vi "mathscrip.vi"(0 "image path":path, 1 "threshoulds array":dbl[](array[numeric]), 5 "error in":errorcluster) -> (12 "imgout":dbl[][](array[numeric]), 13 "error out":errorcluster, 14 "defect ratio 2":dbl, 15 "defect ratio1":dbl, 16 "damage points 2":dbl[][](array[numeric]), 17 "damage points":dbl[][](array[numeric]), 18 "defect type":dbl, 19 "frame statue":dbl)   [LabVIEW 2019]
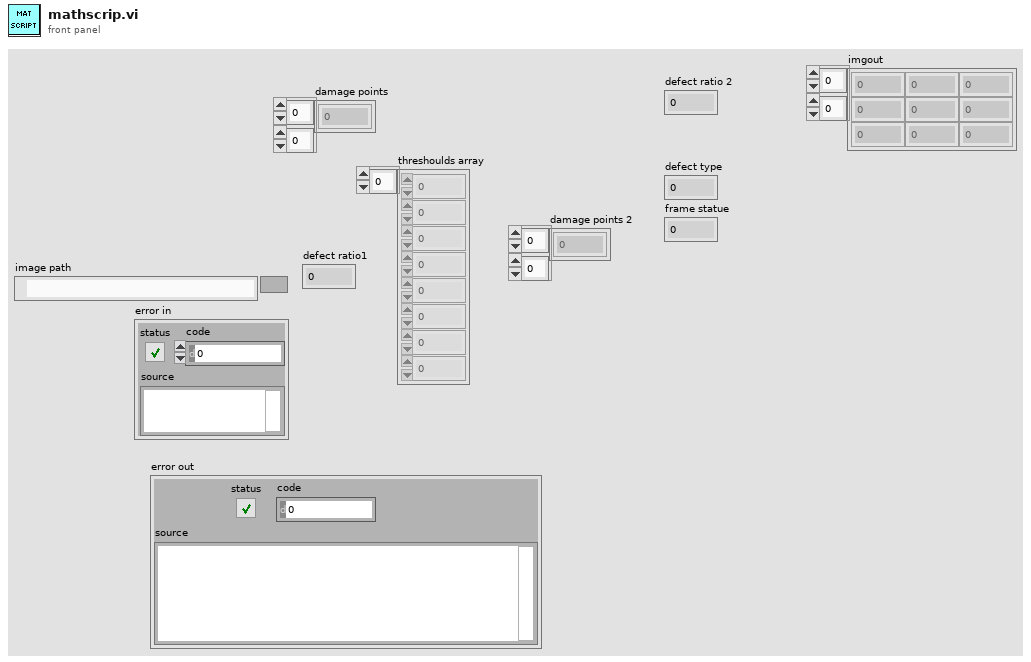
[diagram p1: front panel]
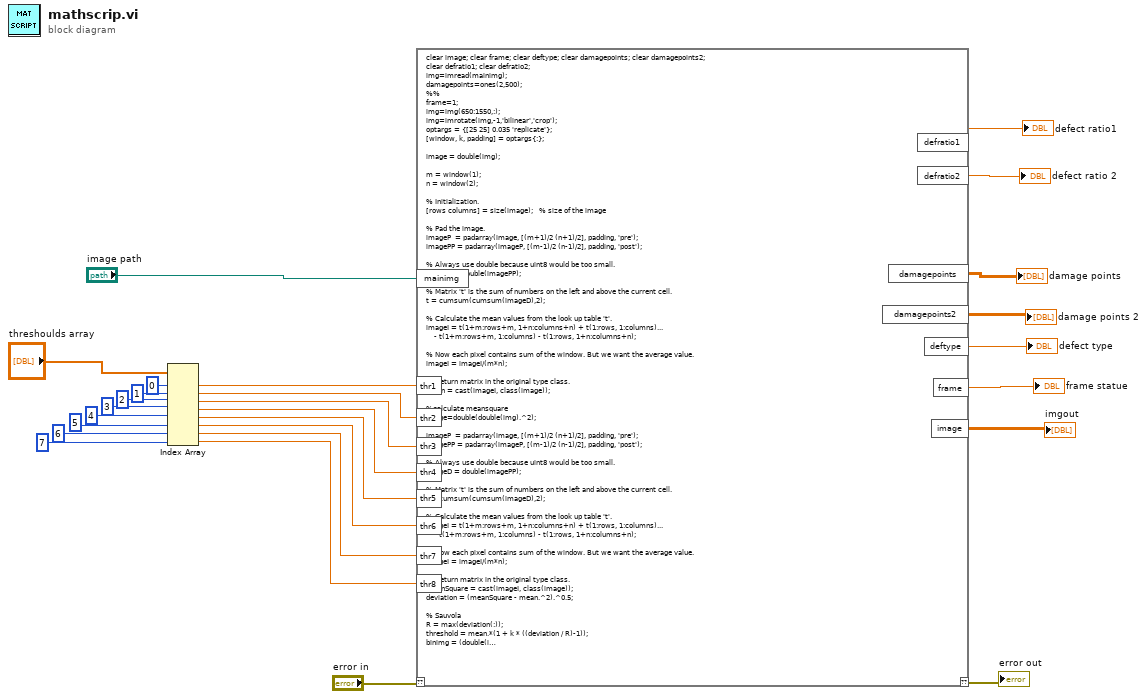
[diagram p0: block diagram]
diagram:
  n1 = Index Array(array="threshoulds array", index #1=0 ("index"), index #2=1 ("index"), index #3=2 ("index"), index #4=3 ("index"), index #5=4 ("index"), index #6=5 ("index"), index #7=6 ("index"), index #8=7 ("index")) -> (element #1=w27:dbl, element #2=w25:dbl, element #3=w24:dbl, element #4=w23:dbl, element #5=w22:dbl, element #6=w21:dbl, element #7=w20:dbl, element #8=w19:dbl)
  n2 = script code="clear image; clear frame; clear deftype; clear damagepoints; clear damagepoints2;\nclear defratio1; clear defratio2;\nimg=imread(mainimg);\ndamagepoints=ones(2,500);\n%%\nframe=1;\nimg=img(650:1550,:);\nimg=imrotate(img,-1,'bilinear','crop');\noptargs = {[25 25] 0.035 'replicate'};\n[window, k, padding] = optargs{:};\n\nimage = double(img);\n\nm = window(1);\nn = window(2);\n\n% Initialization.\n[rows columns] = size(image);   % size of the image\n\n% Pad the image.\nimageP  = padarray(image, [(m+1)/2 (n+1)/2], padding, 'pre');\nimagePP = padarray(imageP, [(m-1)/2 (n-1)/2], padding, 'post');\n\n% Always use double because uint8 would be too small.\nimageD = double(imagePP);\n\n% Matrix 't' is the sum of numbers on the left and above the current cell.\nt = cumsum(cumsum(imageD),2);\n\n% Calculate the mean values from the look up table 't'.\nimageI = t(1+m:rows+m, 1+n:columns+n) + t(1:rows, 1:columns)...\n    - t(1+m:rows+m, 1:columns) - t(1:rows, 1+n:columns+n);\n\n% Now each pixel contains sum of the window. But we want the average value.\nimageI = imageI/(m*n);\n\n% Return matrix in the original type class.\nmean = cast(imageI, class(image));\n\n%calculate meansquare\nimage=double(double(img).^2);\n\nimageP  = padarray(image, [(m+1)/2 (n+1)/2], padding, 'pre');\nimagePP = padarray(imageP, [(m-1)/2 (n-1)/2], padding, 'post');\n\n% Always use double because uint8 would be too small.\nimageD = double(imagePP);\n\n% Matrix 't' is the sum of numbers on the left and above the current cell.\nt = cumsum(cumsum(imageD),2);\n\n% Calculate the mean values from the look up table 't'.\nimageI = t(1+m:rows+m, 1+n:columns+n) + t(1:rows, 1:columns)...\n    - t(1+m:rows+m, 1:columns) - t(1:rows, 1+n:columns+n);\n\n% Now each pixel contains sum of the window. But we want the average value.\nimageI = imageI/(m*n);\n\n% Return matrix in the original type class.\nmeanSquare = cast(imageI, class(image));\ndeviation = (meanSquare - mean.^2).^0.5;\n\n% Sauvola\nR = max(deviation(:));\nthreshold = mean.*(1 + k * ((deviation / R)-1));\nbinimg = (double(img) > threshold);\n%%\n\n%figure,imshow(binimg,[]);\n\ncmplimg=~binimg;\n%cmplimg=cmplimg(70:end-70,:);\n%figure,imshow(cmplimg,[]);\n\nintimg=sum(cmplimg,2)/mean2(cmplimg);\nintimg=max(intimg)-intimg;\n\n%% find the three horizontal line in picture with calculating the horizental integral image  \n                                                             \n[pks,locs] = findpeaks(intimg(1:800),'MINPEAKHEIGHT',4500,'MinPeakDistance',120);\nif numel(pks)<=3                                                             %if there are more than three peaks\n\n    frame=0;\n    defratio1=0;\n    defratio2=0;\n    damagepoints=[];\n    deftype=0;\nelse\n   \n   pks=pks(2:4);\n   locs=locs(2:4);\n\n%% morfing\nh=size(cmplimg,1);\nif locs(1)>170\n    marg1=locs(1)-150;\nelse\n    marg1=20;\nend\n\nif locs(3)<size(cmplimg,1)-190\n    marg2=locs(3)+160;\nelse\n    marg2=size(cmplimg,1)-30;\nend\ncmplimg(1:marg1,:)=0;\ncmplimg(marg2:end,:)=0;\nfor i=1:h\n    cmplimg(i,1:ceil(90+(h-i)*0.17))=0;\n    cmplimg(i,ceil(2150-(h-i)*0.13):end)=0;\nend\n\n\nfor i=1:numel(locs)\n    cmplimg(locs(i)-20:locs(i)+20,:)=0;\nend\n\nse=strel('square',3);\nfo=imopen(cmplimg,se);\n%figure,imshow(fo,[]);\n\nse2=strel('rectangle',[15 1]);\ncmplimg=imclose(fo,se2);\n%figure,imshow(cmplimg,[]);\n\nse3=strel('rectangle',[10 2]);\ncmplimg=imopen(cmplimg,se3);\n%figure,imshow(cmplimg,[]);\n\n\n%%labeling\ncc=bwconncomp(cmplimg);\nl=labelmatrix(cc);\n features=regionprops(cc,'Area','MajorAxisLength','orientation','Centroid');\n% removing the objects that have less than 80 pixel heigth\nidx2=find([features.MajorAxisLength]>80);\ncmplimg=ismember(l,idx2);\n%figure,imshow(cmplimg,[]);\n\ncc=bwconncomp(cmplimg);\n    obnum=cc.NumObjects;\n    l2=labelmatrix(cc);\n    features=regionprops(cc,'Centroid','MajorAxisLength');\n    centr=[features.Centroid];\n    % removing the objects witch are so near to another object. in this method the\n    % objects with smaller height will be removed\n\n    % finding centre of objects\n    k=1:2:numel(centr);\n    xcentr=centr(k);\n    ycentr=centr(k+1);\n    removed=zeros(size(xcentr));\n    % removed matrix: if the object has been removed marked as '2', if only\n    % be close to another object marked as '1';\n    %figure,imshow(l2,[]);\n     for i=1:obnum-1\n         switch i\n\n             case obnum-1\n                 nearobjidx=i+1;\n             case obnum-2 \n                 nearobjidx=i+1:i+2;\n             case obnum-3\n                 nearobjidx=i+1:i+3;\n\n\n             otherwise\n                 nearobjidx=i+1:i+4;\n         end\n                 for j=nearobjidx\n                     xdis=abs(xcentr(i)-xcentr(j));                            % x distance\n                     ydis=abs(ycentr(i)-ycentr(j));                            % y distance\n                     % if the xdis and ydis be less than threshods and not benn\n                     % marked as '1' or '2' \n                     if (xdis<=12 && ydis<=20 && removed(j)==0 && removed(i)==0)\n                         removed(j)=1;\n                         if features(i).MajorAxisLength>features(j).MajorAxisLength\n                             removed(j)=2;\n                         else\n                             removed(i)=2;\n                         end\n\n                     end\n                 end\n\n\n     end\n     % removing the objects witch marked as '2'\n     removidx=find(removed==2);\n     removedobj=ismember(l2,removidx);\n     % final binary image\n     \n     morfimglabel=logical(cmplimg-removedobj);\n   \n      %figure,imshow(morfimglabel);\n     \n     cc=bwconncomp(morfimglabel);\n     objnum=cc.NumObjects;     % number of objects\n    % calculate the area and find the centriod of each object\n    \n   % if objnum>0\n        features=regionprops(cc,'Area','Centroid');\n        area=[features.Area];\n        centr=cat(1,features.Centroid);\n        \n       defthr=zeros(2,objnum);\n       for i=1:objnum\n           if centr(i,2)<locs(1)\n               defthr(1,i)=thr1;\n               defthr(2,i)=thr5;\n           elseif  centr(i,2)<locs(2)\n               defthr(1,i)=thr2;\n               defthr(2,i)=thr6;\n           elseif  centr(i,2)<locs(3)\n               defthr(1,i)=thr3;\n               defthr(2,i)=thr7;\n           else\n               defthr(1,i)=thr4;\n               defthr(2,i)=thr8;\n           end\n       end\n       defind1=find((area>defthr(1,:)));\n       defind2=find(area>defthr(2,:));\n       xdef=round(centr(defind1,1)');\n       ydef=round(centr(defind1,2)');\n       xdef2=round(centr(defind2,1)');\n       ydef2=round(centr(defind2,2)');\n       damagepoints=ones(2,objnum);\n       damagepoints=[xdef;ydef];\n       damagepoints2=[xdef2;ydef2];\n       defratio1=(numel(xdef)/objnum)*100;\n       defratio2=(numel(xdef2)/objnum)*100;\n       if numel(xdef2)>0\n           deftype=2;\n       else\n           deftype=1;\n       end\n\n\n       \n       % figure,imshow(img)\n        \n         %hold on\n        %plot(xdef, ydef, 'r*')\n        %hold off;\nend                                                                         %end off if numel (pks) <3\nclear mainimg;\nclear area; clear binimg; clear cc; \nclear centr; clear cmplimg; clear columns; clear  defind1; clear defind2;\nclear  defthr ; clear deviation; clear features; clear fo; clear h; clear i; clear idx2;\nclear imageD; clear imageI; clear imageP clear imagePP; clear img;\nclear intimg; clear j; clear k; clear l; clear l2; clear locs; clear m; clear marg1; \nclear marg2; clear mean; clear meanSquare; clear morfimglabel; clear n;\nclear nearobjidx; clear objnum; clear obnum; clear optargs; clear padding;\nclear pks; clear R; clear removed; clear removedobj; clear removidx; clear rows;\nclear se; clear se2; clear se3; clear t; clear threshold; clear window; clear xcentr; \nclear xdef; clear xdef2; clear xdis; clear ycentr; clear ydef; clear ydef2; clear ydis;\nclear  thr1; clear thr2; clear thr3; clear thr4; clear thr5; clear thr6; clear thr7; clear thr8;"("??"="error in", "mainimg"="image path", "thr1"=w27, "thr2"=w25, "thr3"=w24, "thr4"=w23, "thr5"=w22, "thr6"=w21, "thr7"=w20, "thr8"=w19) -> ("??"=→"error out":errorcluster, "defratio1"=→"defect ratio1":dbl, "damagepoints"=→"damage points":dbl[][], "defratio2"=→"defect ratio 2":dbl, "damagepoints2"=→"damage points 2":dbl[][], "deftype"=→"defect type":dbl, "frame"=→"frame statue":dbl, "image"=→"imgout":dbl[][])
